vi "Driver Controls.vi"(9 "Arm angle from 'Y'":dbl=86.0 format="%#_13g", 10 "Buttons":bool[](array[boolean]), 11 "POVs":i16[](array[numeric])) -> ()   [LabVIEW 2018]
uses:
  Typedef/XBox Buttons.ctl
  Wrist/Implementation/Wrist Published Globals.vi
  Beak/Implementation/Beak Published Globals.vi
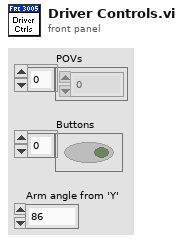
[diagram p1: front panel]
types:
  T1 = typedef "XBox Buttons.ctl" = enum16{"A", "B", "X", "Y", "Left Bumper", "Right Bumper", "Back", "Start", "Left Joystick", "Right Joystick"}
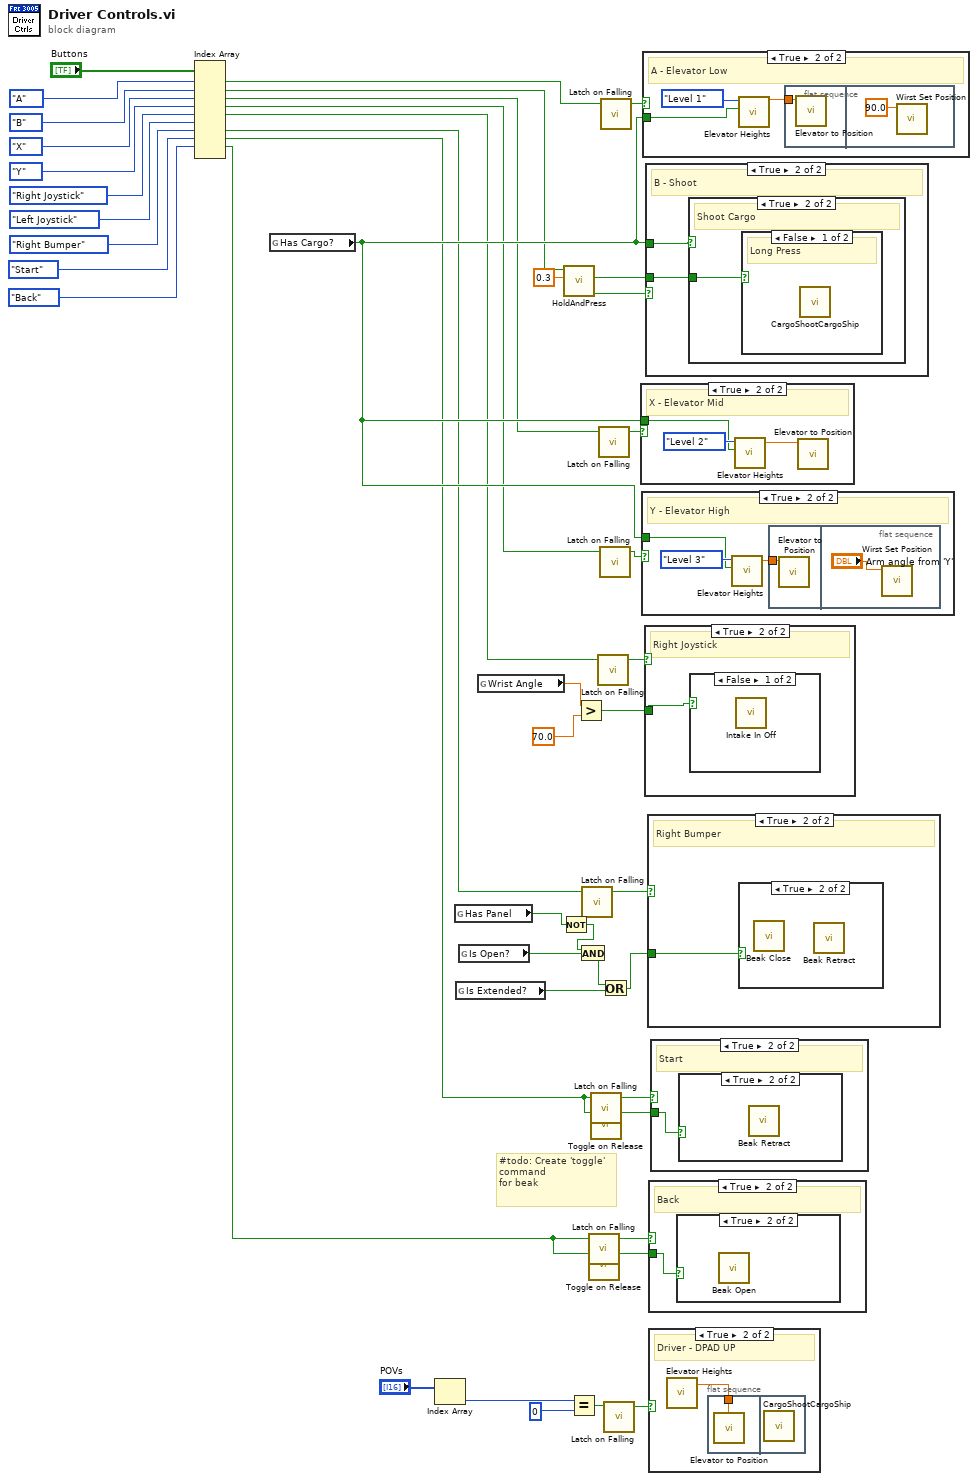
[diagram p0: block diagram]
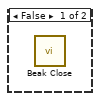
[diagram p5: hidden frame]
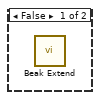
[diagram p7: hidden frame]
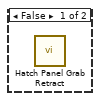
[diagram p9: hidden frame]
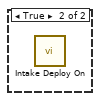
[diagram p11: hidden frame]
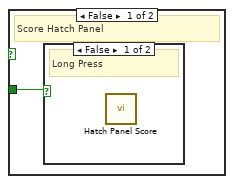
[diagram p13: hidden frame]
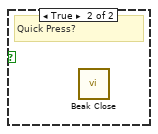
[diagram p14: hidden frame]
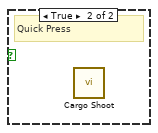
[diagram p15: hidden frame]
diagram:
  # "#todo: Create 'toggle' command\nfor beak"
  n1 = Index Array(array="Buttons", index #1=XBox_Buttons."A" ("Enum"), index #2=XBox_Buttons."B" ("Enum"), index #3=XBox_Buttons."X" ("Enum"), index #4=XBox_Buttons."Y" ("Enum"), index #5=XBox_Buttons."Right Joystick" ("Enum"), index #6=XBox_Buttons."Left Joystick" ("Enum"), index #7=XBox_Buttons."Right Bumper" ("Enum"), index #8=XBox_Buttons."Start" ("Enum"), index #9=XBox_Buttons."Back" ("Enum")) -> (element #1=w8:bool, element #2=w25:bool, element #3=w11:bool, element #4=w12:bool, element #5=w24:bool, element #7=w16:bool, element #8=w20:bool, element #9=w23:bool)  [unwired: 1 in, 2 out]
  n2 = global read "Wrist Published Globals.vi" "Has Cargo?"() -> (w35:bool)
  n3 = Index Array(array="POVs") -> (element=w42:i16)  [unwired: 1 in]
  n4 = global read "Beak Published Globals.vi" "Has Panel"() -> (w31:bool)
  n5 = global read "Beak Published Globals.vi" "Is Extended?"() -> (w30:bool)
  n6 = global read "Beak Published Globals.vi" "Is Open?"() -> (w34:bool)
  n7 = global read "Wrist Published Globals.vi" "Wrist Angle"() -> (w37:dbl)
  n8 = Not(x=w31) -> (.not. x?=w32:bool)
  n9 = call "HoldAndPress.vi"("Holdtime"=0.3, "Input"=w25) -> ("Press?"=w27:bool, "Quick Press"=w28:bool)  [unwired: 4 in, 4 out]
  n10 = Equal?(x=w42, y=0) -> (x = y?=w43:bool)
  n11 = Greater?(x=w37, y=70.0) -> (0:w39:bool)
  n12 = And(x=w32, y=w34) -> (x .and. y?=w33:bool)
  n13 = call "Latch on Falling.vi"("Boolean in"=w16) -> ("Boolean out"=w14:bool)  [unwired: 4 in]
  n14 = call "Latch on Falling.vi"("Boolean in"=w23) -> ("Boolean out"=w22:bool)  [unwired: 4 in]
  n15 = call "Toggle on Release.vi"("Boolean"=w23) -> ("toggle on release"=w21:bool)  [unwired: 10 in]
  n16 = call "Latch on Falling.vi"("Boolean in"=w20) -> ("Boolean out"=w15:bool)  [unwired: 4 in]
  n17 = call "Toggle on Release.vi"("Boolean"=w20) -> ("toggle on release"=w17:bool)  [unwired: 10 in]
  n18 = call "Latch on Falling.vi"("Boolean in"=w24) -> ("Boolean out"=w13:bool)  [unwired: 4 in]
  n19 = call "Latch on Falling.vi"("Boolean in"=w11) -> ("Boolean out"=w10:bool)  [unwired: 4 in]
  n20 = call "Latch on Falling.vi"("Boolean in"=w12) -> ("Boolean out"=w36:bool)  [unwired: 4 in]
  n21 = call "Latch on Falling.vi"("Boolean in"=w8) -> ("Boolean out"=w9:bool)  [unwired: 4 in]
  n22 = Or(x=w33, y=w30) -> (x .or. y?=w29:bool)
  n23 = call "Latch on Falling.vi"("Boolean in"=w43) -> ("Boolean out"=w44:bool)  [unwired: 4 in]
  n24 = case shown="True" w10 {
    tunnel: w35 -> [_ w46]
    frame False {
    }
    frame True {
      # "X - Elevator Mid"
      n25 = call "Elevator Heights.vi"("With Cargo?"=w46, "Level"=enum16{"Level 1", "Level 2", "Level 3"}."Level 2") -> ("Height"=w48:dbl)  [unwired: 8 in, 1 out]
      n26 = call "Elevator to Position.vi"("Elevator Height"=w48) -> ()  [unwired: 10 in, 1 out]
    }
  }
  n27 = case shown="True" w36 {
    tunnel: w35 -> [_ w49]
    frame False {
    }
    frame True {
      # "Y - Elevator High"
      n28 = call "Elevator Heights.vi"("With Cargo?"=w49, "Level"=enum16{"Level 1", "Level 2", "Level 3"}."Level 3") -> ("Height"=w51:dbl)  [unwired: 8 in, 1 out]
      n29 = flat-sequence {
        tunnel: w51 -> [w52]
        frame #0 {
          n30 = call "Elevator to Position.vi"("Elevator Height"=w52) -> ()  [unwired: 10 in, 1 out]
        }
        frame #1 {
          n31 = call "Wirst Set Position.vi"("Setpoint (Degrees)"="Arm angle from 'Y'") -> ()  [unwired: 10 in, 1 out]
        }
      }
    }
  }
  n32 = case shown="True" w9 {
    tunnel: w35 -> [_ w54]
    frame False {
    }
    frame True {
      # "A - Elevator Low"
      n33 = call "Elevator Heights.vi"("With Cargo?"=w54, "Level"=enum16{"Level 1", "Level 2", "Level 3"}."Level 1") -> ("Height"=w56:dbl)  [unwired: 8 in, 1 out]
      n34 = flat-sequence {
        tunnel: w56 -> [w57]
        frame #0 {
          n35 = call "Elevator to Position.vi"("Elevator Height"=w57) -> ()  [unwired: 10 in, 1 out]
        }
        frame #1 {
          n36 = call "Wirst Set Position.vi"("Setpoint (Degrees)"=90.0) -> ()  [unwired: 10 in, 1 out]
        }
      }
    }
  }
  n37 = case shown="True" w13 {
    tunnel: w39 -> [_ w59]
    frame False {
    }
    frame True {
      # "Right Joystick"
      n38 = case shown="False" w59 {
        frame False {
          n39 = call "Intake In Off.vi"() -> ()  [unwired: 11 in, 1 out]
        }
        frame True {
          n40 = call "Intake Deploy On.vi"() -> ()  [unwired: 11 in, 1 out]
        }
      }
    }
  }
  n41 = case shown="True" w27 {
    tunnel: w28 -> [_ w61]
    tunnel: w35 -> [_ w60]
    frame False {
    }
    frame True {
      # "B - Shoot"
      n42 = case shown="True" w60 {
        tunnel: w61 -> [w62 w63]
        frame False {
          # "Score Hatch Panel"
          n43 = case shown="False" w62 {
            frame False {
              # "Long Press"
              n44 = call "Hatch Panel Score.vi"() -> ()  [unwired: 11 in, 1 out]
            }
            frame True {
              # "Quick Press?"
              n45 = call "Beak Close.vi"() -> ()  [unwired: 11 in, 1 out]
            }
          }
        }
        frame True {
          # "Shoot Cargo"
          n46 = case shown="False" w63 {
            frame False {
              # "Long Press"
              n47 = call "CargoShootCargoShip.vi"() -> ()  [unwired: 11 in, 1 out]
            }
            frame True {
              # "Quick Press"
              n48 = call "Cargo Shoot.vi"() -> ()  [unwired: 11 in, 1 out]
            }
          }
        }
      }
    }
  }
  n49 = case shown="True" w14 {
    tunnel: w29 -> [_ w64]
    frame False {
    }
    frame True {
      # "Right Bumper"
      n50 = case shown="True" w64 {
        frame False {
          n51 = call "Hatch Panel Grab Retract.vi"() -> ()  [unwired: 11 in, 1 out]
        }
        frame True {
          n52 = call "Beak Close.vi"() -> ()  [unwired: 11 in, 1 out]
          n53 = call "Beak Retract.vi"() -> ()  [unwired: 11 in, 1 out]
        }
      }
    }
  }
  n54 = case shown="True" w22 {
    tunnel: w21 -> [_ w65]
    frame False {
    }
    frame True {
      # "Back"
      n55 = case shown="True" w65 {
        frame False {
          n56 = call "Beak Close.vi"() -> ()  [unwired: 11 in, 1 out]
        }
        frame True {
          n57 = call "Beak Open.vi"() -> ()  [unwired: 11 in, 1 out]
        }
      }
    }
  }
  n58 = case shown="True" w44 {
    frame False {
    }
    frame True {
      # "Driver - DPAD UP"
      n59 = call "Elevator Heights.vi"() -> ("Cargo Ship Height"=w66:dbl)  [unwired: 10 in, 1 out]
      n60 = flat-sequence {
        tunnel: w66 -> [w67]
        frame #0 {
          n61 = call "Elevator to Position.vi"("Elevator Height"=w67) -> ()  [unwired: 10 in, 1 out]
        }
        frame #1 {
          n62 = call "CargoShootCargoShip.vi"() -> ()  [unwired: 11 in, 1 out]
        }
      }
    }
  }
  n63 = case shown="True" w15 {
    tunnel: w17 -> [_ w68]
    frame False {
    }
    frame True {
      # "Start"
      n64 = case shown="True" w68 {
        frame False {
          n65 = call "Beak Extend.vi"() -> ()  [unwired: 11 in, 1 out]
        }
        frame True {
          n66 = call "Beak Retract.vi"() -> ()  [unwired: 11 in, 1 out]
        }
      }
    }
  }
